vi "Set_K2400_ZeroV.vi"(8 "error in":errorcluster) -> (0 "error out":errorcluster)   [LabVIEW 2020]
panel:
  out "DUTVoltage":dbl
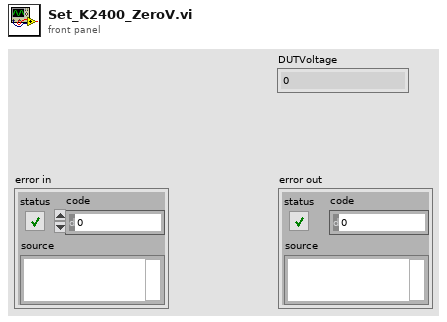
[diagram p1: front panel]
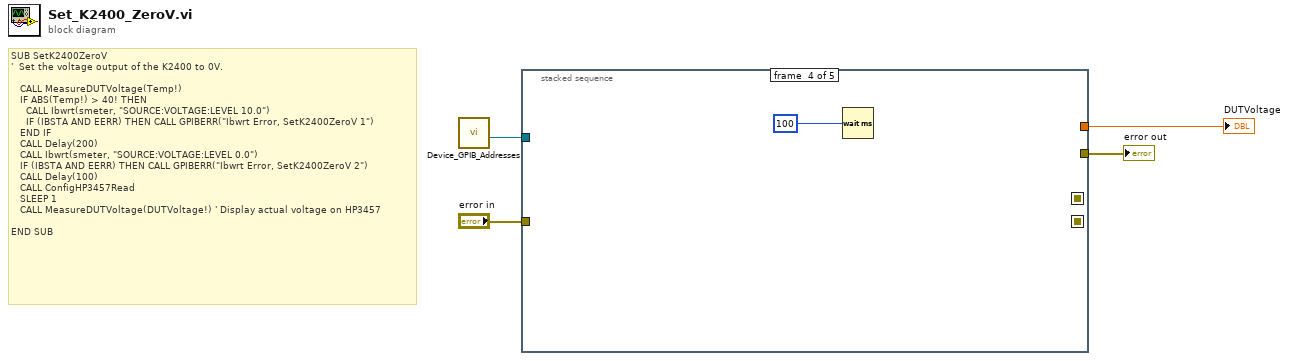
[diagram p0: block diagram]
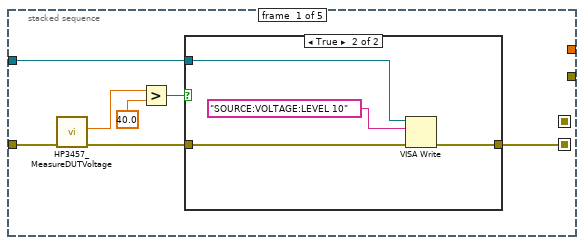
[diagram p2: hidden frame]
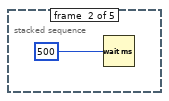
[diagram p4: hidden frame]
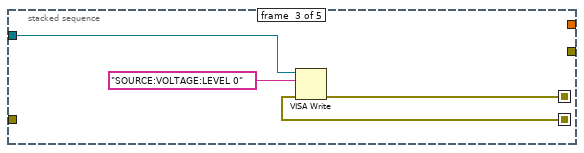
[diagram p5: hidden frame]
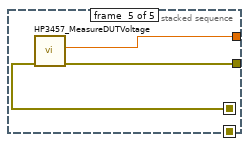
[diagram p6: hidden frame]
diagram:
  # "SUB SetK2400ZeroV\n'  Set the voltage output of the K2400 to 0V.\n\n   CALL MeasureDUTVoltage(Temp!)\n   IF ABS(Temp!) > 40! THEN\n     CALL Ibwrt(smeter, \"SOURCE:VOLTAGE:LEVEL 10.0\")\n     IF (IBSTA AND EERR) THEN CALL GPIBERR(\"Ibwrt Error, SetK2400ZeroV 1\")\n   END IF\n   CALL Delay(200)\n   CALL Ibwrt(smeter, \"SOURCE:VOLTAGE:LEVEL 0.0\")\n   IF (IBSTA AND EERR) THEN CALL GPIBERR(\"Ibwrt Error, SetK2400ZeroV 2\")\n   CALL Delay(100)\n   CALL ConfigHP3457Read\n   SLEEP 1\n   CALL MeasureDUTVoltage(DUTVoltage!) ' Display actual voltage on HP3457\n\nEND SUB"
  n1 = call "Device_GPIB_Addresses.vi"() -> ("HP 4275A Address"=w1:refnum<visa-resource-name>)  [unwired: 9 in, 2 out]
  n2 = stacked-sequence {
    seq-local: [w6 _ _ _ _] -> [_ _ w21 _ _]
    seq-local: [_ _ w20 _ _] -> [_ _ _ _ w23]
    tunnel: [_ _ _ _ w25] -> w4
    tunnel: [_ _ _ _ w24] -> w2
    tunnel: "error in" -> [w10 _ _ _ _]
    tunnel: w1 -> [w5 _ w19 _ _]
    frame #0 {
      n3 = call "HP3457_MeasureDUTVoltage.vi"("error in"=w10) -> ("error out"=w7:errorcluster, "DUTVoltage"=w9:dbl)  [unwired: 8 in]
      n4 = Greater?(x=w9, y=40.0) -> (0:w8:bool)
      n5 = case shown="True" w8 {
        tunnel: w7 -> [w12 w16]
        tunnel: w5 -> [_ w15]
        tunnel: [w12 w14] -> w6
        frame False {
        }
        frame True {
          n6 = VISA Write(VISA resource name=w15, write buffer="SOURCE:VOLTAGE:LEVEL 10", error in (no error)=w16) -> (error out=w14:errorcluster)  [unwired: 2 out]
        }
      }
    }
    frame #1 {
      n7 = Wait (ms)(milliseconds to wait=u32 500) -> ()  [unwired: 1 out]
    }
    frame #2 {
      n8 = VISA Write(VISA resource name=w19, write buffer="SOURCE:VOLTAGE:LEVEL 0", error in (no error)=w21) -> (error out=w20:errorcluster)  [unwired: 2 out]
    }
    frame #3 {
      n9 = Wait (ms)(milliseconds to wait=u32 100) -> ()  [unwired: 1 out]
    }
    frame #4 {
      n10 = call "HP3457_MeasureDUTVoltage.vi"("error in"=w23) -> ("error out"=w25:errorcluster, "DUTVoltage"=w24:dbl)  [unwired: 8 in]
    }
  }
  "error out" <- w4
  "DUTVoltage" <- w2
